vi "Main Sensor Interface.vi"(8 "error in (no error)":errorcluster, 11 "Module_Refs":T2={"ModuleName"=enum."Controller", "Queue"=refnum, "user event"=refnum, "VI Refnum"=refnum, "ShowFP"=FALSE, "StatesTracking Enabled"=FALSE}) -> (0 "error out":errorcluster)   [LabVIEW 2019, in "Sensor Interface.lvlib"]
doc: "Main Module Template of the architecture. Use this as a template to integrate new independent processes into your application."
uses:
  Sensor Interface.lvlib
  Architecture/Typedefs/Module References.ctl
  Architecture/Typedefs/Enum_Module_Name.ctl
  Architecture/Typedefs/Message.ctl
  Typedefs/State Machine Data.ctl
  Typedefs/Config.ctl
  Controller/Typedefs/State Machine States.ctl
  Architecture/Typedefs/Application Configuration.ctl
  Architecture/Modules/Module Template/Typedefs/Config.ctl
  Architecture/Modules/Module Template/SubVIs/Module Template Configuraton Extractor API.vi
  Architecture/Architecture.lvlib
  Architecture/Modules/Module Template/Module Template.lvlib
  Controller/Controller.lvlib
panel:
  in  "User Console":T1
  in  "Stop App":bool
  out "Message":string
  in  "Stop Module":bool
  # "#Architecture\n\nPlace inside this box all visible data."
  # "SENSOR INTERFACE"
  # "[Covers: UI1]"
  # "[Covers: SI1]"
  # "[Covers: UI4]"
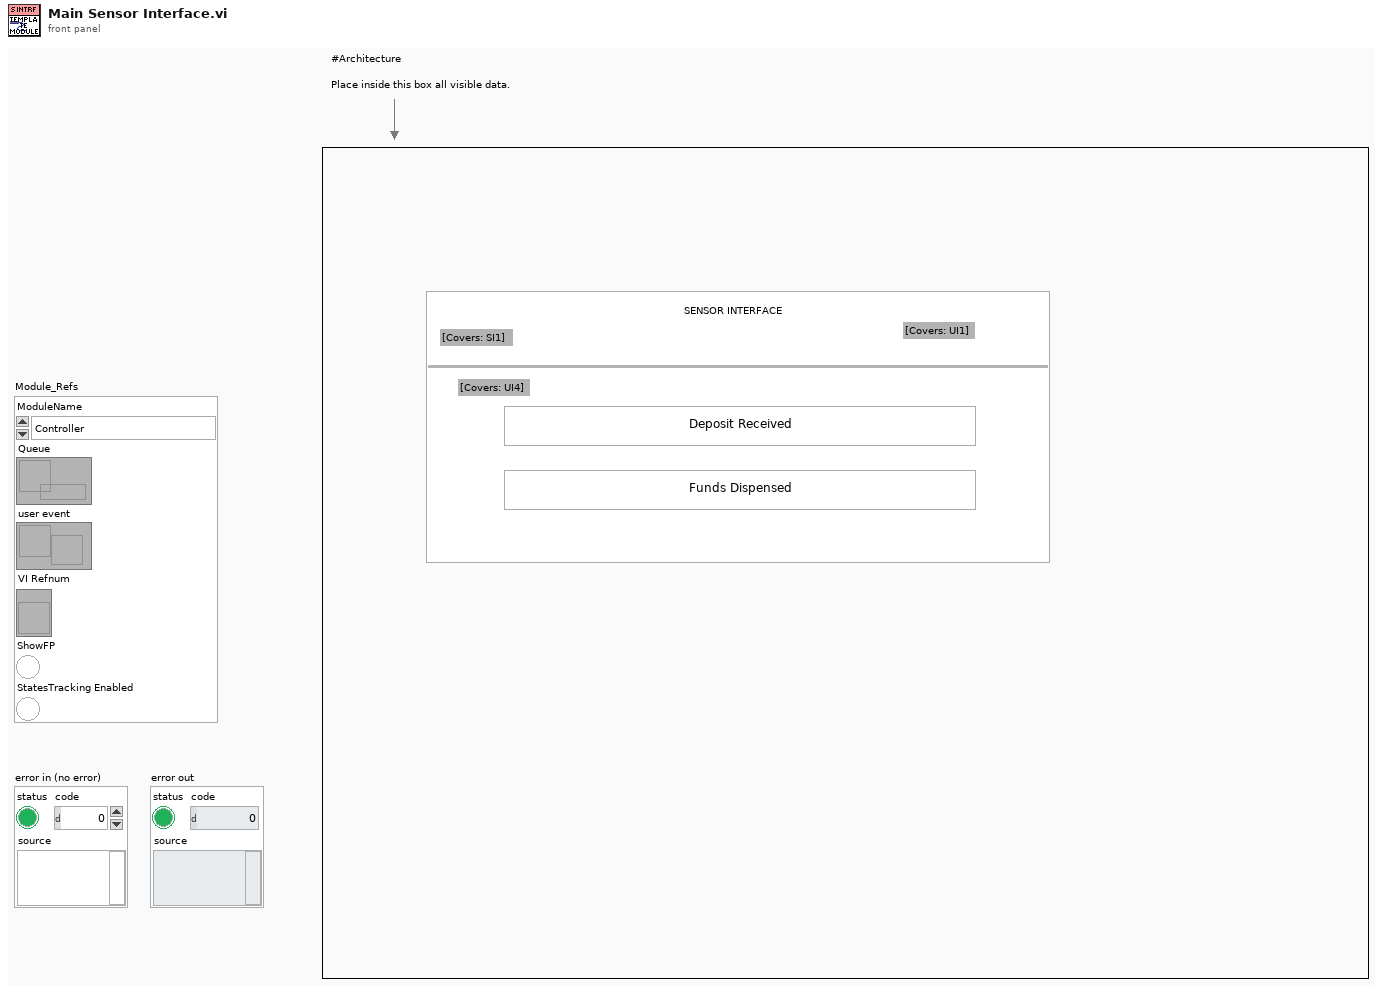
[diagram p1: front panel]
types:
  T1 = cluster{"Deposit Received":bool, "Funds Dispensed":bool}
  T2 = typedef "Architecture.lvlib/Module References.ctl" = cluster{"ModuleName":T3, "Queue":refnum<queue>, "user event":refnum<user-event>, "VI Refnum":refnum<vi>, "ShowFP":bool, "StatesTracking Enabled":bool}
  T3 = typedef "Architecture.lvlib/Enum_Module_Name.ctl" = enum16{"Configuration", "Error_Handler", "Log", "Database", "Controller", "User Console", "Display Console", "Sensor Interface"}
  T4 = typedef "Sensor Interface.lvlib/State Machine Data.ctl" = cluster{"Module_Refs":T2, "Response Data":variant, "Module Template Config":T5}
  T5 = typedef "Sensor Interface.lvlib/Config.ctl" = cluster{"Module Enabled":bool}
  T6 = enum32{"Invalid", "Standard", "Closed", "Hidden", "Minimized", "Maximized"}
  T7 = typedef "Controller.lvlib/State Machine States.ctl" = enum16{"Idle State", "Login State", "Balance Inquiry State", "Deposit State", "Withdrawal State", "Fast Cash State", "Terminate State", "Inactivity Timeout", "Wait For Transaction", "Add Balance"}
  T8 = typedef "Architecture.lvlib/Module Template.lvlib/Config.ctl" = cluster{"Module Enabled":bool}
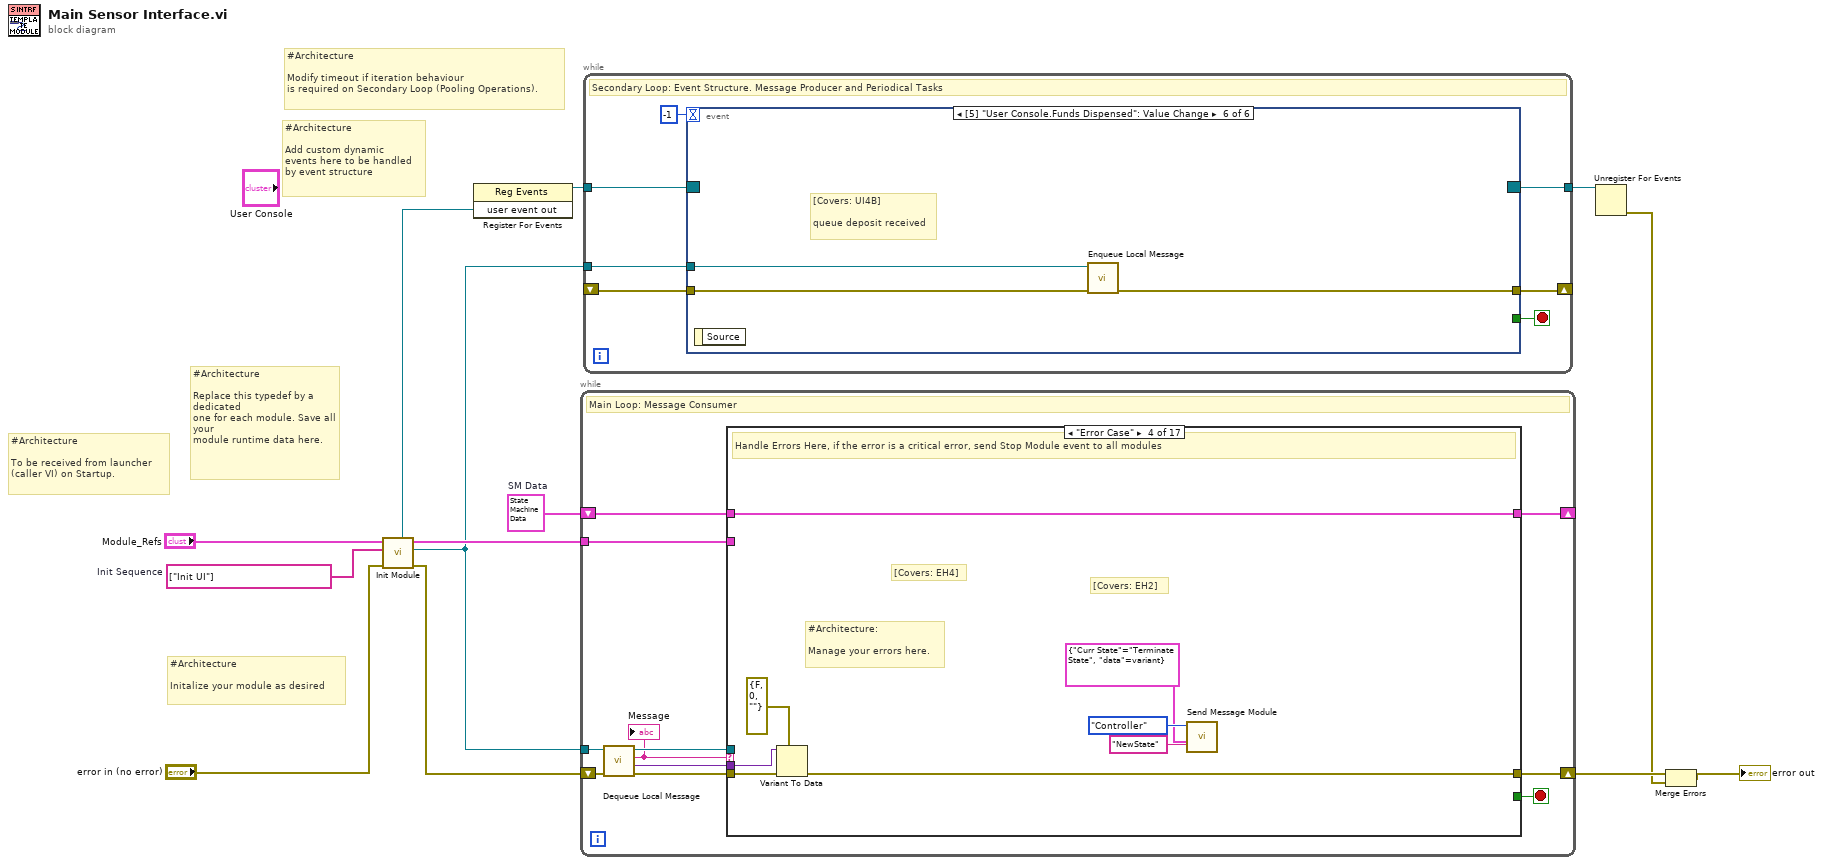
[diagram p0: block diagram]
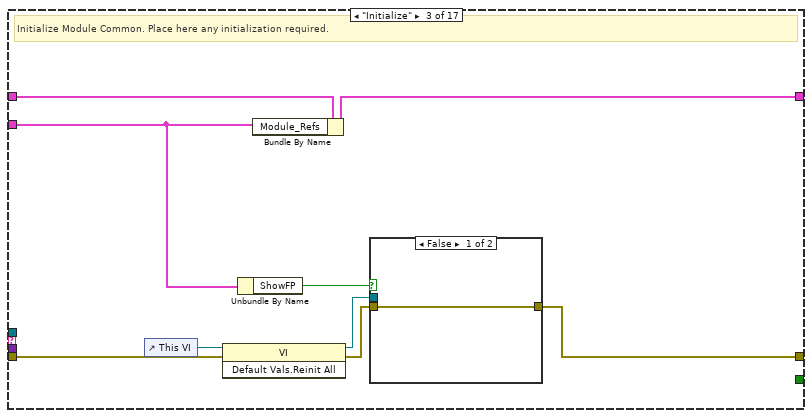
[diagram p4: hidden frame]
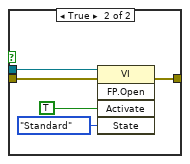
[diagram p5: hidden frame]
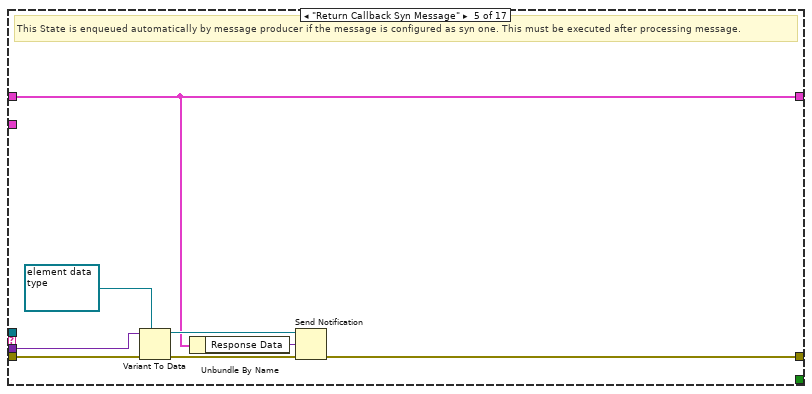
[diagram p6: hidden frame]
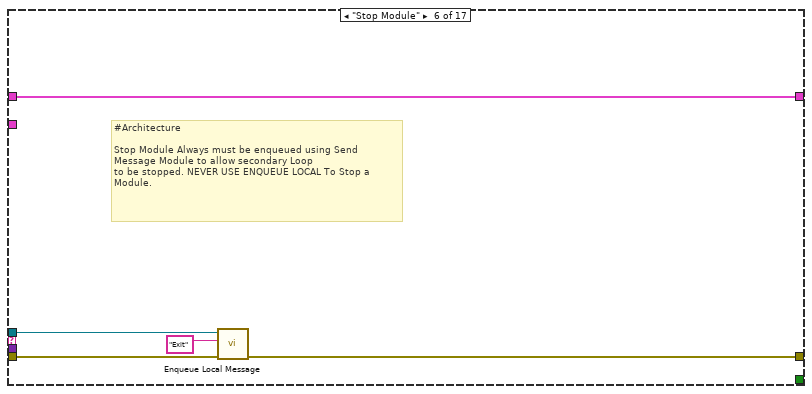
[diagram p7: hidden frame]
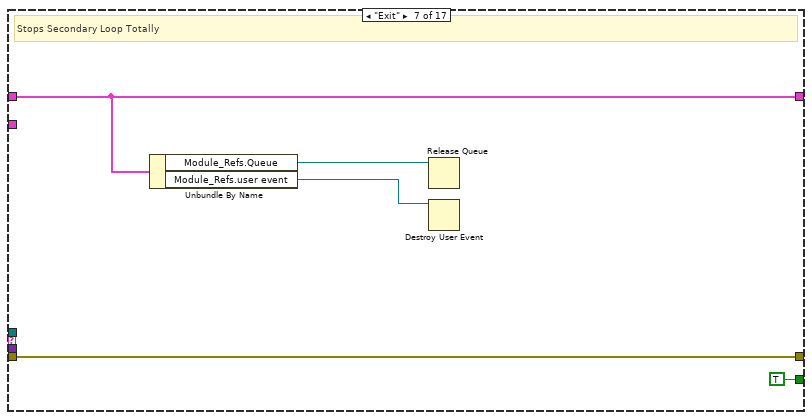
[diagram p8: hidden frame]
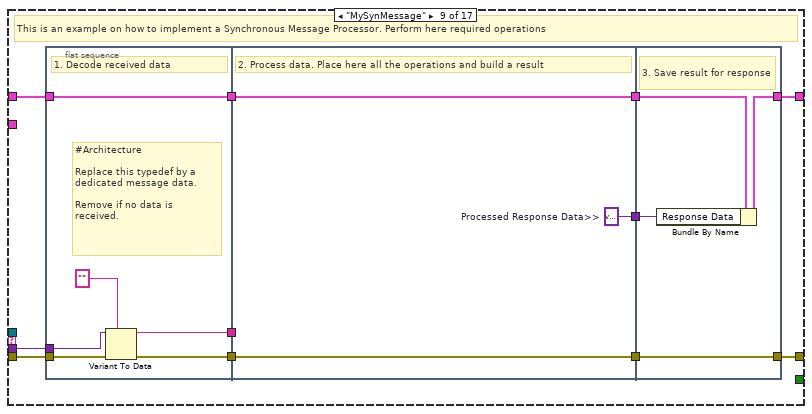
[diagram p10: hidden frame]
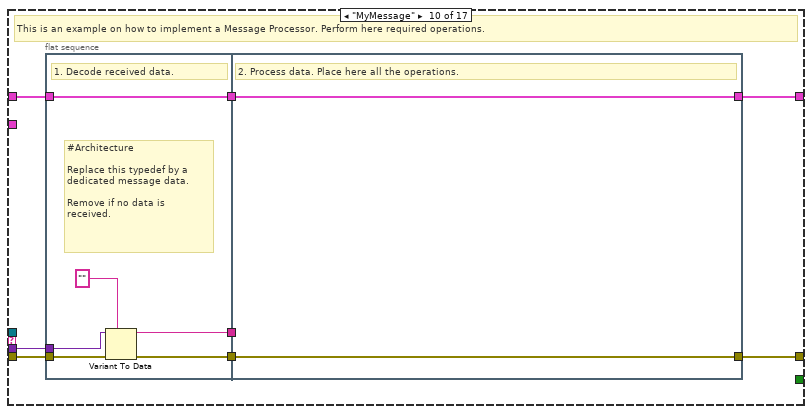
[diagram p11: hidden frame]
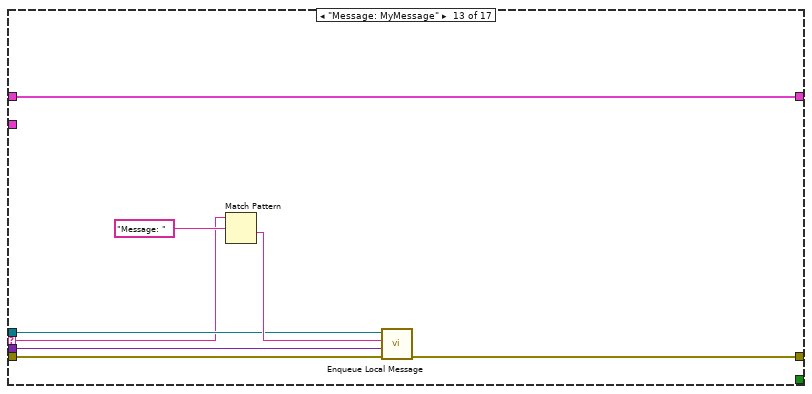
[diagram p14: hidden frame]
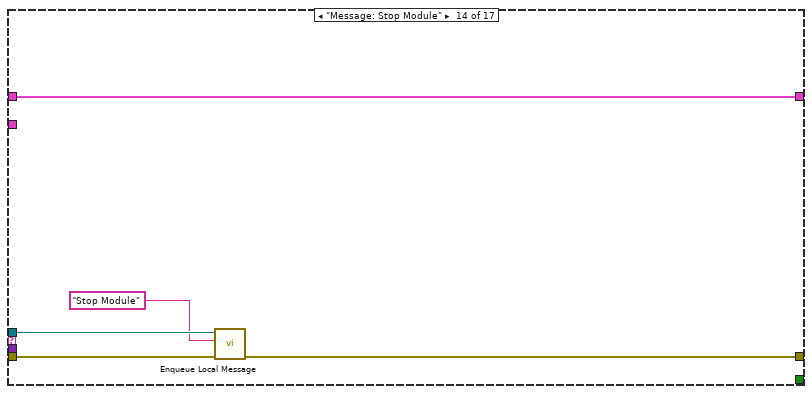
[diagram p15: hidden frame]
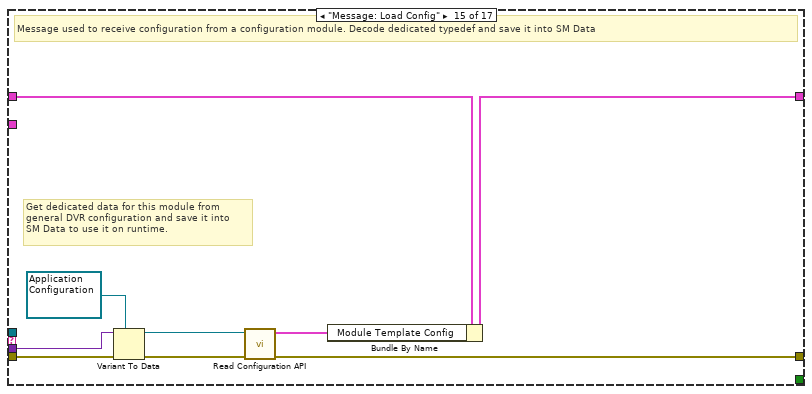
[diagram p16: hidden frame]
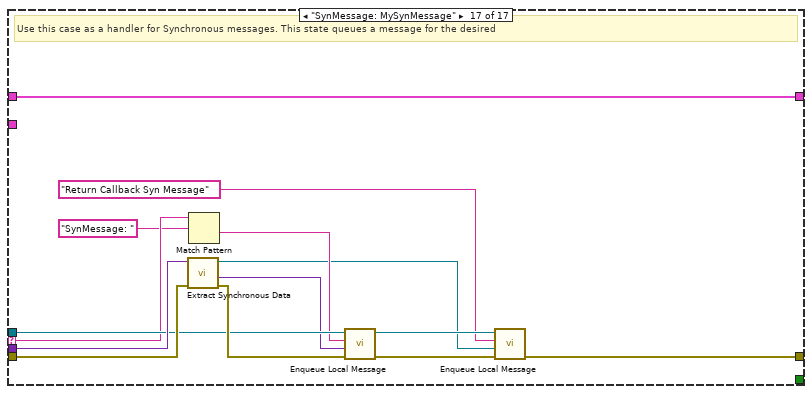
[diagram p18: hidden frame]
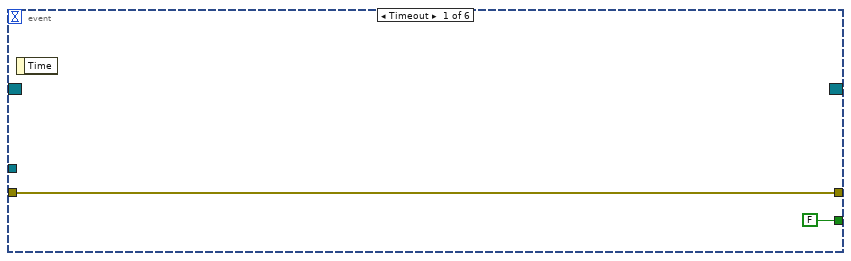
[diagram p19: hidden frame]
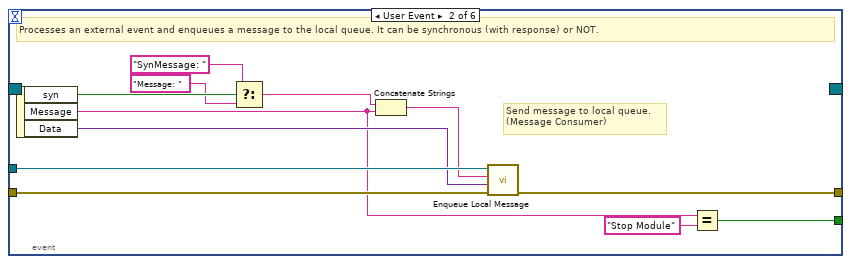
[diagram p20: hidden frame]
diagram:
  w10 = string[] ["Init UI"]  # Init Sequence
  w13 = T4 {"Module_Refs"={"ModuleName"=enum."Controller", "Queue"=refnum, "user event"=refnum, "VI Refnum"=refnum, "ShowFP"=FALSE, "StatesTracking Enabled"=FALSE}, "Response Data"=variant, "Module Template Config"={"Module Enabled"=FALSE}}  # SM Data
  # "#Architecture\n\nModify timeout if iteration behaviour \nis required on Secondary Loop (Pooling Operations)."
  # "#Architecture\n\nAdd custom dynamic \nevents here to be handled \nby event structure"
  # "#Architecture\n\nInitalize your module as desired"
  # "#Architecture\n\nTo be received from launcher \n(caller VI) on Startup."
  # "#Architecture\n\nReplace this typedef by a dedicated \none for each module. Save all your \nmodule runtime data here."
  n1 = call "Init Module.vi"("error in (no error)"="error in (no error)", "Init Sequence"=w10, "Module Refs"="Module_Refs") -> ("error out"=w12:errorcluster, "queue out"=w1:refnum<queue>, "Module Refs Out"=w3:T2, "user event out"=w2:refnum<user-event>)  [unwired: 5 in]
  n2 = register-events(w2) -> (reference out=w9:refnum<event-registration>)  [unwired: 2 in, 1 out]
  n3 = while {
    shift-right: [w23] -> _
    shift-left: w13 -> [w24]
    shift-right: [w22] -> w7
    shift-left: w12 -> [w20]
    tunnel: w1 -> [w21]
    tunnel: w3 -> [w14]
    stop <- w15 stop-if-true
    # "Main Loop: Message Consumer"
    n4 = call "Dequeue Local Message.vi"("error in"=w20, "Msg queue in"=w21) -> ("error out"=w19:errorcluster, "Data"=w16:variant, "Message"=w17:string, "queue out"=w18:refnum<queue>)  [unwired: 6 in]
    "Message" <- w17
    n5 = case shown="\"Error Case\"" w17 {
      selector: w17 -> [_ _ _ _ _ _ _ _ _ _ _ _ w116 _ _ _ w148]
      tunnel: w24 -> [w26 w28 w37 w51 w53 w64 w67 w71 w82 w103 w113 w115 w123 w128 w137 w139 w153]
      tunnel: [w26 w28 w35 w51 w53 w64 w67 w71 w81 w96 w113 w115 w123 w128 w130 w139 w153] -> w23
      tunnel: w19 -> [w25 w27 w36 w50 w59 w63 w69 w70 w75 w99 w112 w114 w120 w127 w136 w138 w152]
      tunnel: [w25 w27 w31 w49 w58 w62 w69 w70 w80 w102 w112 w114 w117 w126 w131 w138 w142] -> w22
      tunnel: w18 -> [_ _ _ _ _ w61 _ _ _ _ _ _ w118 w125 _ _ w149]
      tunnel: w16 -> [_ _ _ w48 w56 _ _ _ w74 w98 _ _ w119 _ w135 _ w150]
      tunnel: [_ _ _ _ _ _ TRUE _ _ _ _ _ _ _ _ _ _] -> w15
      tunnel: w14 -> [_ _ w34 _ _ _ _ _ _ _ _ _ _ _ _ _ _]
      frame "--------State Machine Arquitechture Operations--------" {
      }
      frame "Idle", Default {
        # "Use this state to make iterations if required."
      }
      frame "Initialize" {
        # "Initialize Module Common. Place here any initialization required."
        n6 = control-ref of="This VI"() -> (w29:refnum<vi>)
        n7 = invoke class="VI" method="Default Vals.Reinit All"(reference=w29, error in=w36) -> (reference out=w32:refnum<vi>, error out=w33:errorcluster)  [unwired: 1 in, 1 out]
        n8 = Unbundle By Name(w34) -> ("ShowFP"=w30:bool)
        n9 = Bundle By Name(cluster=w37, "Module_Refs"=w34) -> (w35:T4)
        n10 = case shown="False" w30 {
          tunnel: w33 -> [w38 w43]
          tunnel: [w38 w42] -> w31
          tunnel: w32 -> [_ w41]
          frame False {
          }
          frame True {
            n11 = invoke class="VI" method="FP.Open"(reference=w41, error in=w43, "Activate"=TRUE ("Activate?"), "State"=T6."Standard") -> (error out=w42:errorcluster)  [unwired: 1 in, 4 out]
          }
        }
      }
      frame "Error Case" {
        # "[Covers: EH4]"
        # "[Covers: EH2]"
        # "#Architecture: \n\nManage your errors here."
        # "Handle Errors Here, if the error is a critical error, send Stop Module event to all modules"
        n12 = Variant To Data(error in=w50, type=errorcluster {"status"=FALSE, "code"=0, "source"=""} ("error constant"), Variant=w48) -> (error out=w49:errorcluster)  [unwired: 1 out]
        n13 = call "Send Message Module.vi"("Data"=cluster{"Curr State":T7, "data":variant} {"Curr State"=enum."Terminate State", "data"=variant} ("data"), "Message"="NewState", "Target ModuleName In"=Enum_Module_Name."Controller") -> ()  [unwired: 8 in, 1 out]
      }
      frame "Return Callback Syn Message" {
        # "This State is enqueued automatically by message producer if the message is configured as syn one. This must be executed after processing message."
        n14 = Variant To Data(error in=w59, type=refnum<notifier> refnum ("notifier out"), Variant=w56) -> (data=w54:refnum<notifier>, error out=w57:errorcluster)
        n15 = Unbundle By Name(w53) -> ("Response Data"=w52:variant)
        n16 = Send Notification(notification=w52, notifier=w54, error in (no error)=w57) -> (error out=w58:errorcluster)  [unwired: 1 out]
      }
      frame "Stop Module" {
        # "#Architecture\n\nStop Module Always must be enqueued using Send Message Module to allow secondary Loop\nto be stopped. NEVER USE ENQUEUE LOCAL To Stop a Module."
        n17 = call "Enqueue Local Message.vi"("error in"=w63, "Message"="Exit", "Msg queue in"=w61) -> ("error out"=w62:errorcluster)  [unwired: 7 in, 1 out]
      }
      frame "Exit" {
        # "Stops Secondary Loop Totally"
        n18 = Unbundle By Name(w67) -> ("Module_Refs.Queue"=w66:refnum<queue>, "Module_Refs.user event"=w65:refnum<user-event>)
        n19 = Release Queue(queue=w66) -> ()  [unwired: 2 in, 3 out]
        n20 = Destroy User Event(user event=w65) -> ()  [unwired: 1 in, 1 out]
      }
      frame "--------------State Machine Custom States-------------" {
      }
      frame "MySynMessage" {
        # "This is an example on how to implement a Synchronous Message Processor. Perform here required operations"
        n21 = flat-sequence {
          tunnel: w75 -> [w86]
          tunnel: w82 -> [w88]
          tunnel: [w88] -> w79
          tunnel: [w84] -> w78
          tunnel: w74 -> [w85]
          tunnel: [w83] -> w73
          tunnel: w79 -> [w91]
          tunnel: w78 -> [w90]
          tunnel: [w91] -> w77
          tunnel: [w90] -> w76
          tunnel: w73 -> [_]
          tunnel: [w89] -> w72
          tunnel: [w94] -> w80
          tunnel: [w93] -> w81
          tunnel: w77 -> [w95]
          tunnel: w76 -> [w94]
          tunnel: w72 -> [w92]
          frame #0 {
            # "#Architecture\n\nReplace this typedef by a dedicated message data.\n\nRemove if no data is received."
            # "1. Decode received data"
            n22 = Variant To Data(error in=w86, type="", Variant=w85) -> (data=w83:string, error out=w84:errorcluster)
          }
          frame #1 {
            w89 = variant  # Processed Response Data>>
            # "2. Process data. Place here all the operations and build a result"
          }
          frame #2 {
            # "3. Save result for response"
            n23 = Bundle By Name(cluster=w95, "Response Data"=w92) -> (w93:T4)
          }
        }
      }
      frame "MyMessage" {
        # "This is an example on how to implement a Message Processor. Perform here required operations."
        n24 = flat-sequence {
          tunnel: w99 -> [w107]
          tunnel: w103 -> [w109]
          tunnel: [w109] -> w101
          tunnel: [w105] -> w100
          tunnel: w98 -> [w106]
          tunnel: [w104] -> w97
          tunnel: w101 -> [w110]
          tunnel: w100 -> [w111]
          tunnel: w97 -> [_]
          tunnel: [w111] -> w102
          tunnel: [w110] -> w96
          frame #0 {
            # "#Architecture\n\nReplace this typedef by a dedicated message data.\n\nRemove if no data is received."
            # "1. Decode received data."
            n25 = Variant To Data(error in=w107, type="", Variant=w106) -> (data=w104:string, error out=w105:errorcluster)
          }
          frame #1 {
            # "2. Process data. Place here all the operations."
          }
        }
      }
      frame "Init UI" {
        # "[Covers: IS3]\n\nPlace here all calls to property nodes to \ninitialize UI controls and Indicators.\n\nAll controls are disabled"
      }
      frame "--------------Dynamic Events Messages----------------" {
      }
      frame "Message: MyMessage" {
        n26 = Match Pattern(string=w116, regular expression="Message: ") -> (after substring=w121:string)  [unwired: 1 in, 3 out]
        n27 = call "Enqueue Local Message.vi"("error in"=w120, "Data"=w119, "Message"=w121, "Msg queue in"=w118) -> ("error out"=w117:errorcluster)  [unwired: 6 in, 1 out]
      }
      frame "Message: Stop Module" {
        n28 = call "Enqueue Local Message.vi"("error in"=w127, "Message"="Stop Module", "Msg queue in"=w125) -> ("error out"=w126:errorcluster)  [unwired: 7 in, 1 out]
      }
      frame "Message: Load Config" {
        # "Get dedicated data for this module from \ngeneral DVR configuration and save it into \nSM Data to use it on runtime."
        # "Message used to receive configuration from a configuration module. Decode dedicated typedef and save it into SM Data"
        n29 = Variant To Data(error in=w136, type=refnum<data-value> refnum ("data value reference"), Variant=w135) -> (data=w133:refnum<data-value>, error out=w132:errorcluster)
        n30 = call-poly "Read Configuration API.vi"("error constant"=w132, "General Config DVR In"=w133) -> ("error out"=w131:errorcluster, "Module Template Config"=w129:T8)  [unwired: 8 in]
        n31 = Bundle By Name(cluster=w137, "Module Template Config"=w129) -> (w130:T4)
      }
      frame "------------Synchronous Event Messages--------------" {
      }
      frame "SynMessage: MySynMessage" {
        # "Use this case as a handler for Synchronous messages. This state queues a message for the desired"
        n32 = call "Extract Synchronous Data.vi"("error in 2"=w152, "Variant"=w150) -> ("error in"=w151:errorcluster, "Data Out"=w145:variant, "notifier out"=w140:refnum<notifier>)  [unwired: 7 in]
        n33 = Match Pattern(string=w148, regular expression="SynMessage: ") -> (after substring=w146:string)  [unwired: 1 in, 3 out]
        n34 = call "Enqueue Local Message.vi"("error in"=w151, "Data"=w145, "Message"=w146, "Msg queue in"=w149) -> ("error out"=w144:errorcluster, "queue out"=w143:refnum<queue>)  [unwired: 6 in]
        n35 = call "Enqueue Local Message.vi"("error in"=w144, "Data"=w140, "Message"="Return Callback Syn Message", "Msg queue in"=w143) -> ("error out"=w142:errorcluster)  [unwired: 6 in, 1 out]
      }
    }
  }
  n36 = while {
    tunnel: w9 -> [w160]
    tunnel: w1 -> [w157]
    tunnel: [w156] -> w8
    shift-right: [w154] -> _
    shift-left: _ -> [w155]
    stop <- w158 stop-if-true
    # "Secondary Loop: Event Structure. Message Producer and Periodical Tasks"
    n37 = event shown="[5] \"User Console.Funds Dispensed\": Value Change" {
      selector: w160 -> [_ _ _ _ _ _]
      dyn-events: [_ _ _ _ _ _] -> w156
      timeout: -1 -> [_ _ _ _ _ _]
      tunnel: [FALSE w169 TRUE _ _ _] -> w158
      tunnel: w157 -> [_ w174 w176 _ w184 w187]
      tunnel: w155 -> [w161 w173 w179 w181 w186 w189]
      tunnel: [w161 w172 w177 w180 w185 w188] -> w154
      event Timeout {
        n38 = event-data() -> ()  [unwired: 1 in, 1 out]
      }
      event User Event {
        # "Send message to local queue. \n(Message Consumer)"
        # "Processes an external event and enqueues a message to the local queue. It can be synchronous (with response) or NOT."
        n39 = event-data() -> ("syn"=w166:bool, "Message"=w168:string, "Data"=w171:variant)  [unwired: 1 in]
        n40 = Select(t="SynMessage: " ("string"), s=w166, f="Message: " ("string")) -> (s? t:f=w163:string)
        n41 = Concatenate Strings(w163, w168) -> (w170:string)
        n42 = call "Enqueue Local Message.vi"("error in"=w173, "Data"=w171, "Message"=w170, "Msg queue in"=w174) -> ("error out"=w172:errorcluster)  [unwired: 6 in, 1 out]
        n43 = Equal?(x=w168, y="Stop Module") -> (x = y?=w169:bool)
      }
      event "Stop Module": Value Change {
        n44 = event-data() -> ()  [unwired: 1 in, 1 out]
        n45 = call "Enqueue Local Message.vi"("error in"=w179, "Message"="Stop Module", "Msg queue in"=w176) -> ("error out"=w177:errorcluster)  [unwired: 7 in, 1 out]
      }
      event "Stop App": Value Change {
        w183 = TRUE  # All Modules
        # "Send Stop To All Modules"
        n46 = event-data() -> ()  [unwired: 1 in, 1 out]
        n47 = call "Send Message Modules.vi"("All Modules"=w183, "Error In"=w181, "Message"="Stop Module") -> ("error in (no error)"=w180:errorcluster)  [unwired: 8 in]
      }
      event "User Console.Deposit Received": Value Change {
        # "[Covers: UI4A] \n\nqueue deposit received"
        n48 = event-data() -> ()  [unwired: 1 in, 1 out]
        n49 = call "Enqueue Local Message.vi"("error in"=w186, "Msg queue in"=w184) -> ("error out"=w185:errorcluster)  [unwired: 8 in, 1 out]
      }
      event "User Console.Funds Dispensed": Value Change {
        # "[Covers: UI4B] \n\nqueue deposit received"
        n50 = event-data() -> ()  [unwired: 1 in, 1 out]
        n51 = call "Enqueue Local Message.vi"("error in"=w189, "Msg queue in"=w187) -> ("error out"=w188:errorcluster)  [unwired: 8 in, 1 out]
      }
    }
  }
  n52 = Unregister For Events(event registration refnum=w8) -> (error out=w6:errorcluster)  [unwired: 1 in]
  n53 = Merge Errors(w7, w6) -> (→"error out":errorcluster)
